vi "Channel Status.vi"(8 "Error In":errorcluster, 10 "Channel (0)":i32, 11 "VISA resource name":refnum<visa-resource-name>) -> (0 "Error Out":errorcluster, 1 "Status Bits":T1, 2 "Status":u16 format="%.0x", 3 "dup VISA resource name":refnum<visa-resource-name>)   [LabVIEW 2011, in "MGC647C.lvlib"]
doc: "Read status of a channel."
uses:
  <instrlib>/MGC647C/MGC647C.lvlib
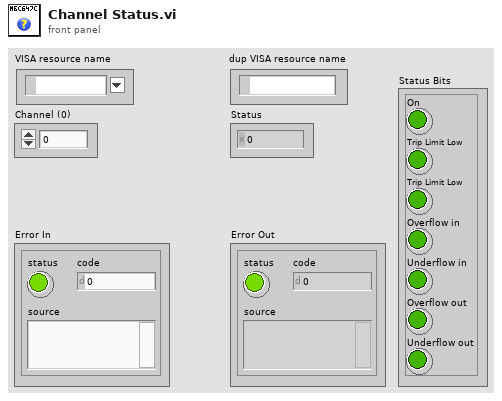
[diagram p1: front panel]
types:
  T1 = cluster{"On":bool, "Boolean array[1]":bool, "Boolean array[2]":bool, "Boolean array[3]":bool, "Trip Limit Low":bool, "Trip Limit Low":bool, "Overflow in":bool, "Underflow in":bool, "Overflow out":bool, "Underflow out":bool, "Boolean array[10]":bool, "Boolean array[11]":bool, "Boolean array[12]":bool, "Boolean array[13]":bool, "Boolean array[14]":bool, "Boolean array[15]":bool}
  T2 = cluster{"Boolean array[0]":bool, "Boolean array[1]":bool, "Boolean array[2]":bool, "Boolean array[3]":bool, "Boolean array[4]":bool, "Boolean array[5]":bool, "Boolean array[6]":bool, "Boolean array[7]":bool, "Boolean array[8]":bool, "Boolean array[9]":bool, "Boolean array[10]":bool, "Boolean array[11]":bool, "Boolean array[12]":bool, "Boolean array[13]":bool, "Boolean array[14]":bool, "Boolean array[15]":bool}
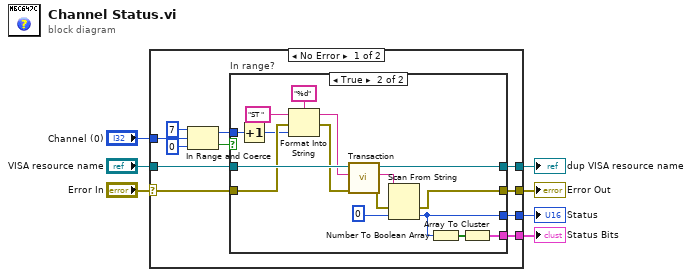
[diagram p0: block diagram]
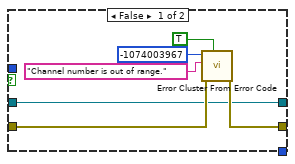
[diagram p2: hidden frame]
diagram:
  n1 = case shown="No Error" "Error In" {
    selector: "Error In" -> [w15 w42]
    tunnel: "VISA resource name" -> [w18 w41]
    tunnel: [w17 w41] -> w6
    tunnel: [w16 w42] -> w5
    tunnel: "Channel (0)" -> [w12 _]
    tunnel: [w9 _] -> w2
    tunnel: [w8 _] -> w1
    frame No Error {
      n2 = In Range and Coerce(upper limit=7, x=w12, lower limit=0) -> (coerced(x)=w11:i32, In Range?=w10:bool)
      n3 = case "In range?" shown="True" w10 {
        tunnel: w18 -> [w22 w40]
        tunnel: [w22 w39] -> w17
        tunnel: [w23 w29] -> w16
        tunnel: w15 -> [w24 w38]
        tunnel: w11 -> [_ w36]
        tunnel: [_ w27] -> w9
        tunnel: [_ w25] -> w8
        frame False {
          n4 = call <vilib>:"Error Cluster From Error Code.vi"("show call chain? (False)"=TRUE, "error in (no error)"=w24, "error message (\"\")"="Channel number is out of range." ("error message (\"\")"), "error code (0)"=-1074003967) -> ("error out"=w23:errorcluster)  [unwired: 5 in]
        }
        frame True {
          n5 = Increment(x=w36) -> (x+1=w35:i32)
          n6 = Format Into String(format string="%d", initial string="ST ", error in=w38, w35) -> (resulting string=w34:string, error out=w37:errorcluster)
          n7 = call <instrlib>:"Transaction.vi"("Error In"=w37, "Command"=w34, "VISA resource name"=w40) -> ("Error Out"=w30:errorcluster, "Response"=w31:string, "dup VISA resource name"=w39:refnum<visa-resource-name>)  [unwired: 6 in]
          n8 = Scan From String(input string=w31, error in=w30, default 1=u16 0 ("Numeric Indicator")) -> (error out=w29:errorcluster, output 1=w27:u16)  [unwired: 2 in, 2 out]
          n9 = Number To Boolean Array(number=w27) -> (Boolean array=w26:bool[])
          n10 = Array To Cluster(array=w26) -> (cluster=w25:T2)
        }
      }
    }
    frame Error {
    }
  }
  "dup VISA resource name" <- w6
  "Error Out" <- w5
  "Status" <- w2
  "Status Bits" <- w1
